vi "AnalysisCommand.vi"(10 "Command":string="UU\u0001\u0005\u001cþÿà") -> (0 "DataOut":u8[](array[numeric]), 1 "CMD":u8, 2 "ID":u8)   [LabVIEW 2013]
panel:
  out "Length":u8
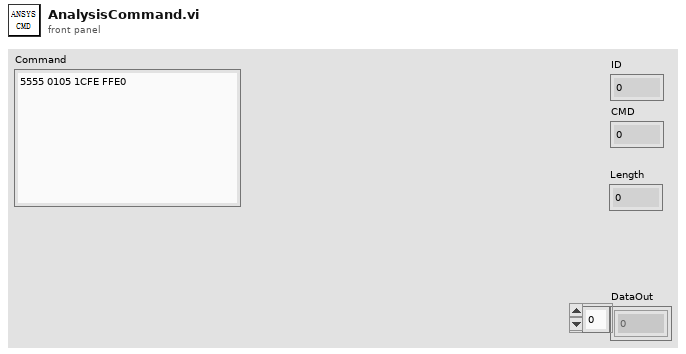
[diagram p1: front panel]
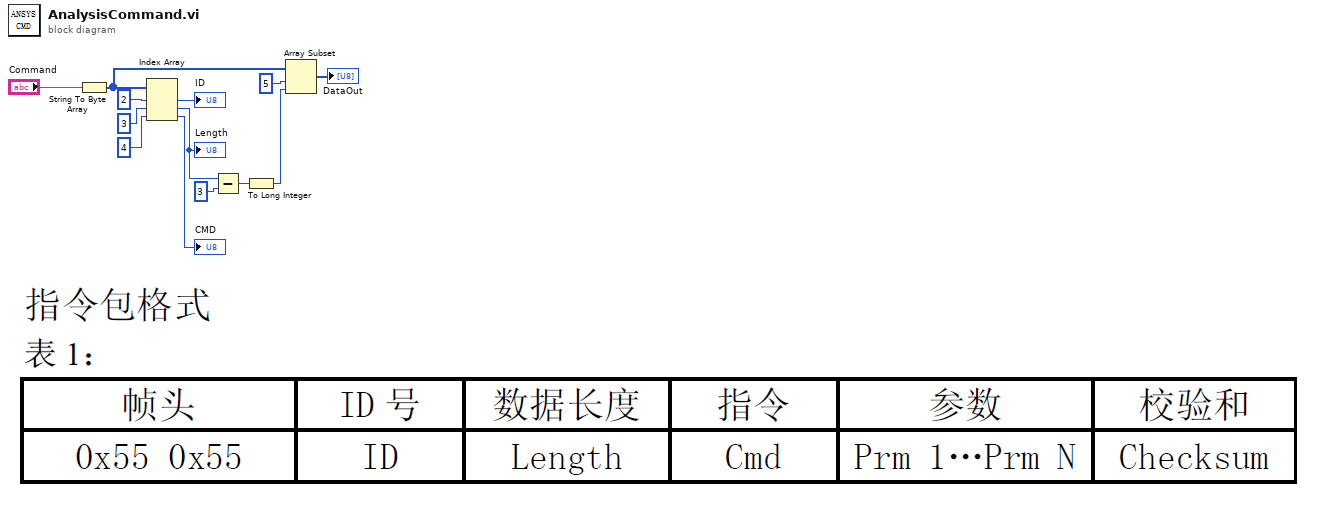
[diagram p0: block diagram]
diagram:
  n1 = String To Byte Array(string="Command") -> (unsigned byte array=w5:u8[])
  n2 = Index Array(array=w5, index #1=2 ("index"), index #2=3 ("index"), index #3=4 ("index")) -> (element #1=→"ID":u8, element #2=w7:u8, element #3=→"CMD":u8)
  "Length" <- w7
  n3 = Subtract(x=w7, y=u8 3) -> (x-y=w3:u8)
  n4 = To Long Integer(number=w3) -> (32bit integer=w2:i32)
  n5 = Array Subset(array=w5, index=5, length=w2) -> (→"DataOut":u8[])
